vi "Initialize User Interface.vi"(8 "error in (no error)":errorcluster, 11 "Car Wash Console in":refnum<class "Car Wash Console.lvclass">) -> (0 "error out":errorcluster, 3 "Car Wash Console out":refnum<class "Car Wash Console.lvclass">)   [LabVIEW 2016, in "CLD Exam - Car Wash.lvlib" / "Car Wash Console.lvclass"]
uses:
  Car Wash Console.lvclass
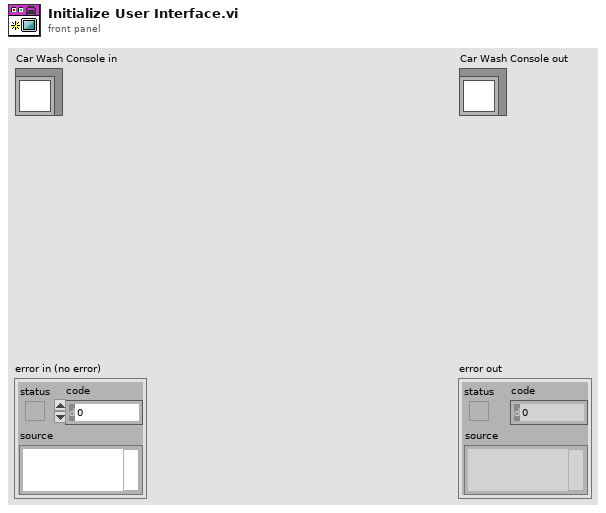
[diagram p1: front panel]
types:
  T1 = enum8{"Enabled", "Disabled", "Disabled and Grayed Out"}
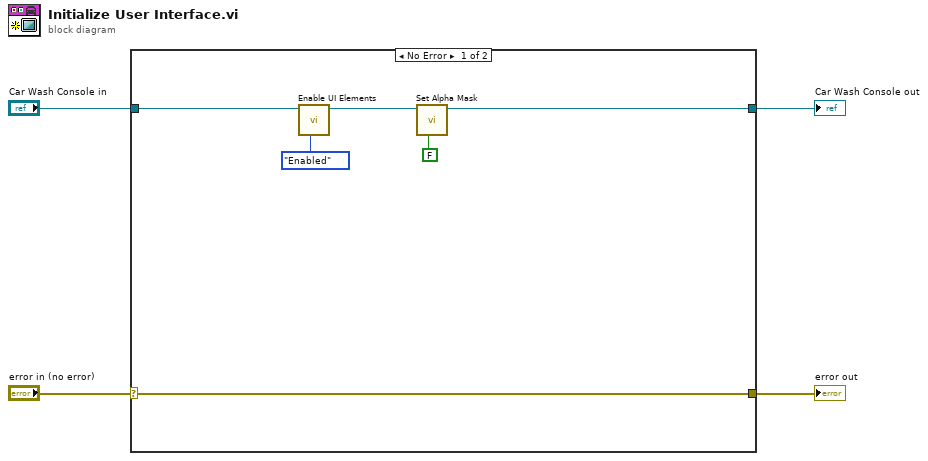
[diagram p0: block diagram]
diagram:
  n1 = case shown="No Error" "error in (no error)" {
    selector: "error in (no error)" -> [w10 w12]
    tunnel: [w10 w12] -> w3
    tunnel: [w8 w11] -> w1
    tunnel: "Car Wash Console in" -> [w7 w11]
    frame No Error {
      n2 = call "Enable UI Elements.vi"("Disabled"=T1."Enabled", "Car Wash Console in"=w7) -> ("Car Wash Console out"=w6:refnum<class "Car Wash Console.lvclass">)  [unwired: 9 in]
      n3 = call "Set Alpha Mask.vi"("Mask?"=FALSE ("Visible"), "Car Wash Console in"=w6) -> ("Car Wash Console out"=w8:refnum<class "Car Wash Console.lvclass">)  [unwired: 8 in, 1 out]
    }
    frame Error {
    }
  }
  "error out" <- w3
  "Car Wash Console out" <- w1
